vi "zad_5_read.vi"() -> ()   [LabVIEW 2025]
panel:
  in  "error in":errorcluster
  out "error out":errorcluster
  out "String":string
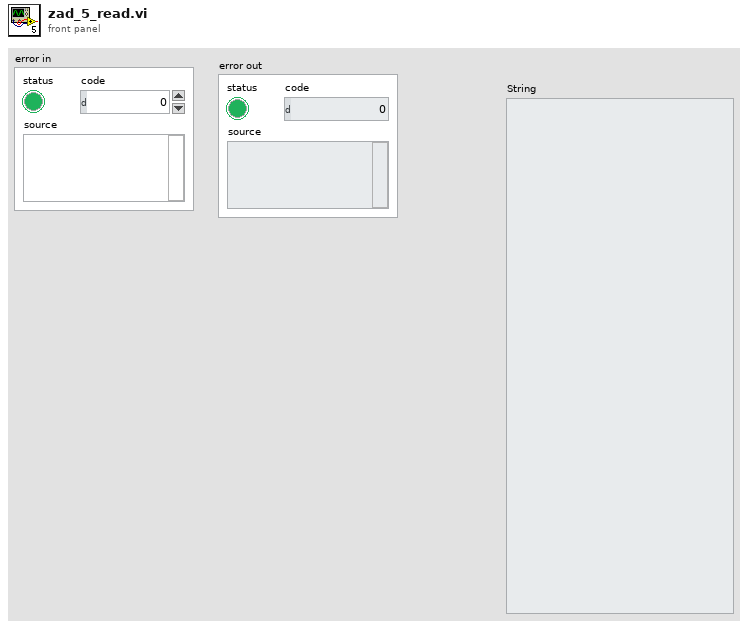
[diagram p1: front panel]
types:
  T1 = enum16{"open", "replace", "create", "open or create", "replace or create", "replace or create with confirmation"}
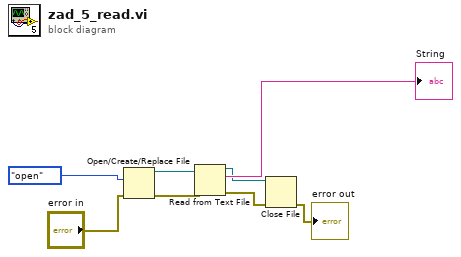
[diagram p0: block diagram]
diagram:
  n1 = Open/Create/Replace File(error in="error in", operation (0:open)=T1."open") -> (refnum out=w1:refnum<file>, error out=w5:errorcluster)  [unwired: 4 in, 1 out]
  n2 = Read from Text File(file (use dialog)=w1, error in=w5) -> (refnum out=w2:refnum<file>, text=→"String":string, error out=w7:errorcluster)  [unwired: 2 in, 1 out]
  n3 = Close File(refnum=w2, error in=w7) -> (error out=→"error out":errorcluster)  [unwired: 1 out]
